vi "Occupancy Grid Generation.vi"() -> ()   [LabVIEW 2017]
uses:
  <vilib>/Analysis/NI_AALPro.lvlib
  <vilib>/robotics/Navigation/shared/WorldMap/OccupancyGridWorldMap/NI_Robotics_OccupancyGridWorldMap.lvclass
panel:
  out "path":cluster{"X":i32, "Y":i32}[](array[cluster])
  in  "endPos":cluster{"x":i32, "y":i32}={"x"=0, "y"=6}
  in  "curPos":cluster{"x":i32, "y":i32}
  out "Frequency":u32=10
  in  "Resolution":dbl=50.0
  out "Intensity Graph":dbl[][](graph)
  in  "Y position":dbl=5000.0
  in  "X position":dbl=5000.0
  in  "stop":bool
  out "XY Graph":cluster{dbl[], dbl[]}(graph)
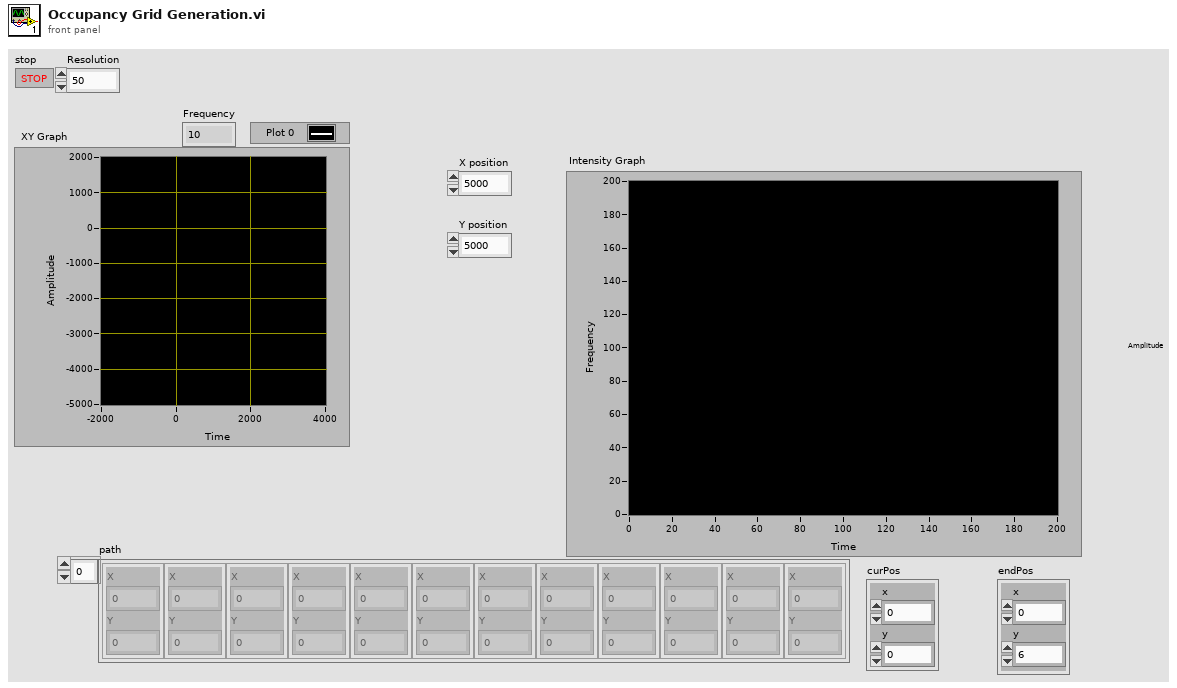
[diagram p1: front panel]
types:
  T1 = typedef "LidarPoint.ctl" = cluster{"X":dbl, "Y":dbl}
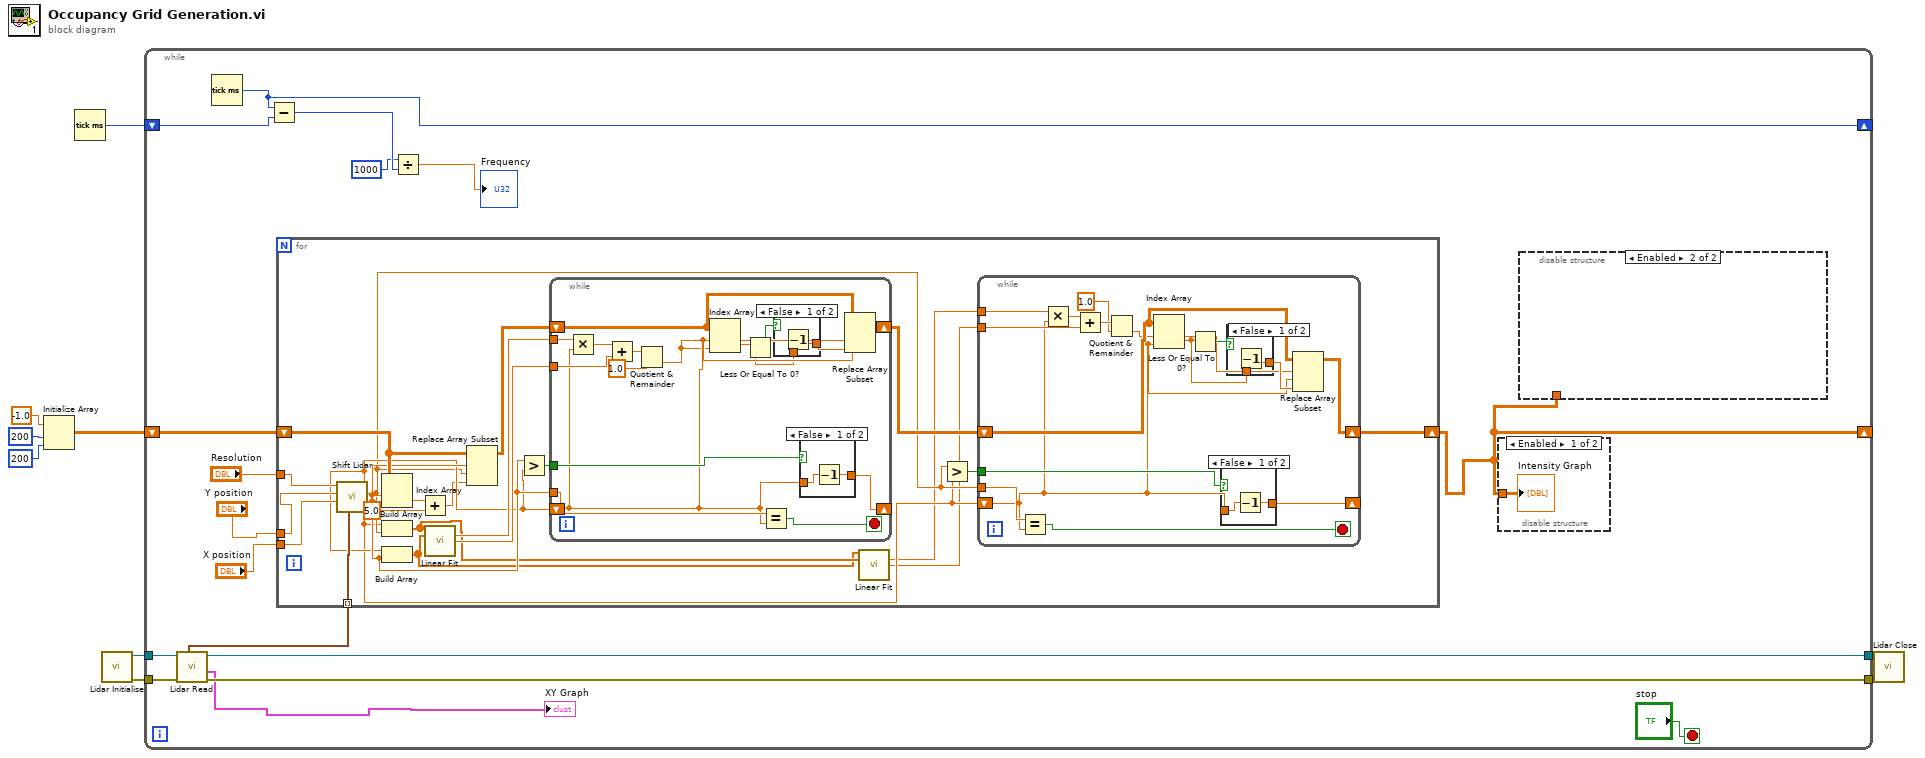
[diagram p0: block diagram]
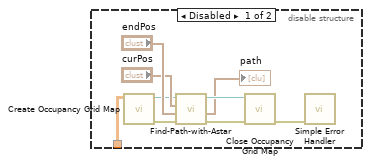
[diagram p2: hidden frame]
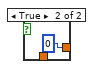
[diagram p4: hidden frame]
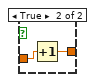
[diagram p5: hidden frame]
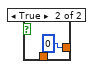
[diagram p6: hidden frame]
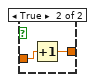
[diagram p7: hidden frame]
diagram:
  n1 = Initialize Array(-1.0 ("element"), 200 ("dimension size"), 200 ("dimension size")) -> (w3:dbl[][])
  n2 = Tick Count (ms)() -> (millisecond timer value=w1:u32)
  n3 = call "Lidar Initialise.vi"() -> ("error out"=w8:errorcluster, "VISA resource name out"=w9:refnum<visa-resource-name>)  [unwired: 10 in]
  n4 = while {
    tunnel: w9 -> [w26]
    tunnel: w8 -> [w25]
    tunnel: [w24] -> w7
    tunnel: [w23] -> w6
    shift-right: [w12] -> _
    shift-left: w3 -> [w18]
    shift-right: [w15] -> _
    shift-left: w1 -> [w17]
    stop <- "stop" stop-if-true
    n5 = call "Lidar Read.vi"("error in (no error)"=w25, "VISA resource name"=w26) -> ("error out"=w23:errorcluster, "Visual Out"=→"XY Graph":cluster{dbl[], dbl[]}, "VISA resource name out"=w24:refnum<visa-resource-name>, "XYflipped"=w10:T1[])  [unwired: 2 in, 3 out]
    n6 = Tick Count (ms)() -> (millisecond timer value=w15:u32)
    n7 = Subtract(x=w15, y=w17) -> (x-y=w14:u32)
    n8 = for {
      tunnel: "Y position" -> [w57]
      tunnel: "X position" -> [w50]
      tunnel: "Resolution" -> [w59]
      tunnel: w10 -> [w58] mode=indexing
      shift-right: [w44] -> w12
      shift-left: w18 -> [w56]
      n9 = call "Shift Lidar.vi"("XY"=w58, "X position"=w50, "Y position"=w57, "Resolution"=w59) -> ("PosY"=w42:dbl, "Shifted X"=w53:dbl, "Shifted Y"=w43:dbl, "PosX"=w49:dbl)  [unwired: 4 in]
      n10 = Index Array(array=w56, index (row)=w53, index (col)=w43) -> (element=w48:dbl)
      n11 = Build Array(w42, w43) -> (w40:dbl[])
      n12 = Build Array(w49, w53) -> (w39:dbl[])
      n13 = Add(x=w48, y=5.0) -> (x+y=w47:dbl)
      n14 = call <vilib>:"Linear Fit.vi"("Y"=w40, "X"=w39) -> ("slope"=w55:dbl, "intercept"=w54:dbl)  [unwired: 9 in, 3 out]
      n15 = Replace Array Subset(array=w56, new element=w47, index (row)=w53, index (col)=w43) -> (w51:dbl[][])
      n16 = Greater?(x=w53, y=w49) -> (0:w52:bool)
      n17 = while {
        tunnel: w53 -> [w97]
        shift-right: [w95] -> _
        shift-left: w49 -> [w90]
        tunnel: w55 -> [w94]
        tunnel: w54 -> [w92]
        tunnel: w52 -> [w96]
        shift-right: [w89] -> w45
        shift-left: w51 -> [w91]
        stop <- w98 stop-if-true
        n18 = Multiply(x=w94, y=w90) -> (x*y=w93:dbl)
        n19 = Add(x=w93, y=w92) -> (x+y=w85:dbl)
        n20 = Quotient & Remainder(x=w85, y=1.0) -> (floor(x/y)=w83:dbl)  [unwired: 1 out]
        n21 = Index Array(array=w91, index (row)=w90, index (col)=w83) -> (element=w86:dbl)
        n22 = Less Or Equal To 0?(x=w86) -> (x <= 0?=w88:bool)
        n23 = Equal?(x=w97, y=w90) -> (x = y?=w98:bool)
        n24 = case shown="False" w88 {
          tunnel: [w100 0] -> w87
          tunnel: w86 -> [w99 _]
          frame False {
            n25 = Decrement(x=w99) -> (x-1=w100:dbl)
          }
          frame True {
          }
        }
        n26 = case shown="False" w96 {
          tunnel: w90 -> [w102 w105]
          tunnel: [w103 w104] -> w95
          frame False {
            n27 = Decrement(x=w102) -> (x-1=w103:dbl)
          }
          frame True {
            n28 = Increment(x=w105) -> (x+1=w104:dbl)
          }
        }
        n29 = Replace Array Subset(array=w91, new element=w87, index (row)=w90, index (col)=w83) -> (w89:dbl[][])
      }
      n30 = call <vilib>:"Linear Fit.vi"("Y"=w39, "X"=w40) -> ("slope"=w38:dbl, "intercept"=w37:dbl)  [unwired: 9 in, 3 out]
      n31 = Greater?(x=w43, y=w42) -> (0:w41:bool)
      n32 = while {
        shift-right: [w64] -> w44
        shift-left: w45 -> [w63]
        shift-right: [w72] -> _
        shift-left: w42 -> [w61]
        tunnel: w43 -> [w74]
        tunnel: w41 -> [w73]
        tunnel: w38 -> [w71]
        tunnel: w37 -> [w69]
        stop <- w75 stop-if-true
        n33 = Equal?(x=w74, y=w61) -> (x = y?=w75:bool)
        n34 = Multiply(x=w71, y=w61) -> (x*y=w70:dbl)
        n35 = Add(x=w70, y=w69) -> (x+y=w68:dbl)
        n36 = Quotient & Remainder(x=w68, y=1.0) -> (floor(x/y)=w60:dbl)  [unwired: 1 out]
        n37 = Index Array(array=w63, index (row)=w60, index (col)=w61) -> (element=w65:dbl)
        n38 = Less Or Equal To 0?(x=w65) -> (x <= 0?=w66:bool)
        n39 = case shown="False" w73 {
          tunnel: w61 -> [w79 w82]
          tunnel: [w80 w81] -> w72
          frame False {
            n40 = Decrement(x=w79) -> (x-1=w80:dbl)
          }
          frame True {
            n41 = Increment(x=w82) -> (x+1=w81:dbl)
          }
        }
        n42 = case shown="False" w66 {
          tunnel: [w77 0] -> w62
          tunnel: w65 -> [w76 _]
          frame False {
            n43 = Decrement(x=w76) -> (x-1=w77:dbl)
          }
          frame True {
          }
        }
        n44 = Replace Array Subset(array=w63, new element=w62, index (row)=w60, index (col)=w61) -> (w64:dbl[][])
      }
    }
    n45 = Divide(x=u32 1000 ("y"), y=w14) -> (x/y=→"Frequency":dbl)
    n46 = disable-structure shown="Enabled" {
      disable-tunnel: w12 -> [w36 _]
      frame Enabled {
        "Intensity Graph" <- w36
      }
      frame Disabled {
      }
    }
    n47 = disable-structure shown="Enabled" {
      disable-tunnel: w12 -> [w27 _]
      frame Disabled {
        n48 = call <vilib>:"Create Occupancy Grid Map.vi"("occupancy grid"=w27) -> ("error out"=w35:errorcluster, "map reference out"=w32:refnum<data-value>)  [unwired: 9 in]
        n49 = call "Find-Path-with-Astar.vi"("error in (no error)"=w35, "goal node"="endPos", "start node"="curPos", "map reference in"=w32) -> ("error out"=w30:errorcluster, "Array"=→"path":cluster{"X":i32, "Y":i32}[], "map reference out"=w31:refnum<data-value>)  [unwired: 5 in]
        n50 = call <vilib>:"Close Occupancy Grid Map.vi"("error in (no error)"=w30, "map reference in"=w31) -> ("error out"=w29:errorcluster)  [unwired: 9 in]
        n51 = call <vilib>:"Simple Error Handler.vi"("error in (no error)"=w29) -> ()  [unwired: 4 in, 5 out]
      }
      frame Enabled {
      }
    }
  }
  n52 = call "Lidar Close.vi"("error in (no error)"=w6, "VISA resource name"=w7) -> ()  [unwired: 9 in, 1 out]
